vi "XY Graph Set Style of Selected Plots.vi"(8 "Error In":errorcluster, 9 "Plot Style":T2={"Plot Style"=enum."unchanged", "Histogram Type"=enum."Left Bound", "Line Tickness"=enum."unchanged", "Line Style"=enum."unchanged", "Point Style"=enum."Small Filled Square", "Line Color"=0, "Point Color"=0, "Anti-aliased"=FALSE, "Line Color Chooser"=enum."unchanged", "Point Color Chooser"=enum."unchanged", "Line Color List"="", "Point Color List"=""}, 11 "XYGraph Ref":T1) -> (0 "Error Out":errorcluster, 1 "Message":string, 3 "XYGraph Ref":T1, 5 "Graph Caption or Label":string)   [LabVIEW 2021, in "XY Graph Add-Ons.lvlib"]
uses:
  XY Graph Add-Ons.lvlib
  XY Graph Refnum.ctl
  Plot Style 3.ctl
  Graphs.lvlib
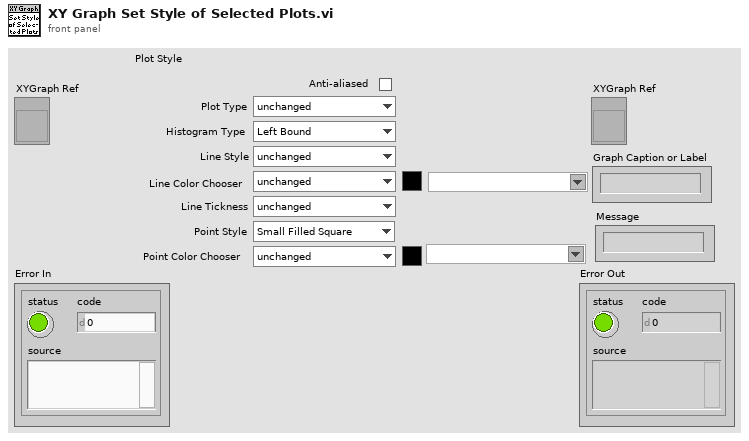
[diagram p1: front panel]
types:
  T1 = typedef "XY Graph Add-Ons.lvlib/XY Graph Refnum.ctl" = refnum<vi>
  T2 = typedef "Graphs.lvlib/Plot Style 3.ctl" = cluster{"Plot Style":enum16{"unchanged", "Line", "Symbol", "Line + Symbol", "Histogram", "Histogram + Symbol"}, "Histogram Type":enum16{"unchanged", "Left Bound", "Center", "Right Bound"}, "Line Tickness":enum16{"unchanged", "Thin", "1 pixel", "2 pixel", "3 pixel", "4 pixel", "5 pixel"}, "Line Style":enum16{"unchanged", "Plain", "Long Dash", "Short Dash", "Long-Short Dash", "Long-Short-Short Dash"}, "Point Style":enum16{"unchanged", "None", "Empty Circle", "Filled Circle", "Thick Circle", "Dotted Circle", "Empty Square", "Filled Square", "Thick Square", "Dotted Square", "Small Filled Square", "Dot", "Cross", "Tiny Cross", "Large X", "Small x", "Diamond", "Small Empty Square"}, "Line Color":u32, "Point Color":u32, "Anti-aliased":bool, "Line Color Chooser":enum16{"unchanged", "Color Box", "Color List"}, "Point Color Chooser":enum16{"unchanged", "Color Box", "Color List"}, "Line Color List":string, "Point Color List":string}
  T3 = typedef "Graphs.lvlib/Single Plot Style 2.ctl" = cluster{"Plot Style":enum16{"unchanged", "Line", "Symbol", "Line + Symbol", "Histogram", "Histogram + Symbol"}, "Histogram Type":enum16{"unchanged", "Left Bound", "Center", "Right Bound"}, "Line Tickness":enum16{"unchanged", "Thin", "1 pixel", "2 pixel", "3 pixel", "4 pixel", "5 pixel"}, "Line Style":enum16{"unchanged", "Plain", "Long Dash", "Short Dash", "Long-Short Dash", "Long-Short-Short Dash"}, "Point Style":enum16{"unchanged", "None", "Empty Circle", "Filled Circle", "Thick Circle", "Dotted Circle", "Empty Square", "Filled Square", "Thick Square", "Dotted Square", "Small Filled Square", "Dot", "Cross", "Tiny Cross", "Large X", "Small x", "Diamond", "Small Empty Square"}, "Line Color":u32, "Line Color defined?":bool, "Point Color":u32, "Point Color defined?":bool, "Anti-aliased":bool}
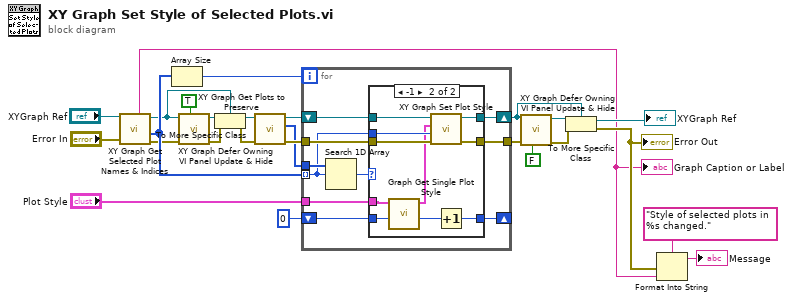
[diagram p0: block diagram]
diagram:
  n1 = call "XY Graph Get Selected Plot Names & Indices.vi"("error in (no error)"="Error In", "XYGraph in"="XYGraph Ref") -> ("error out"=w21:errorcluster, "Selected Plots"=w25:i32[], "XYGraph out"=w12:T1, "Graph Name"=w1:string)  [unwired: 5 in, 1 out]
  "Graph Caption or Label" <- w1
  n2 = Array Size(array=w25) -> (size(s)=w24:i32)
  n3 = call "XY Graph Defer Owning VI Panel Update & Hide.vi"("Defer Owning Panel Update"=TRUE, "error in (no error)"=w21, "XY Graph Refnum in"=w12) -> ("error out"=w11:errorcluster)  [unwired: 7 in, 1 out]
  n4 = To More Specific Class(target class=w12, reference=w12, error in=w11) -> (specific class reference=w7:T1, error out=w6:errorcluster)
  n5 = call "XY Graph Get Plots to Preserve.vi"("Error In"=w6, "XYGraph in"=w7) -> ("Error Out"=w5:errorcluster, "Preserved Plots"=w3:i32[], "XYGraph dup"=w4:T1)  [unwired: 6 in, 1 out]
  n6 = for {
    N: w24 -> [_]
    tunnel: w3 -> [w31]
    tunnel: w25 -> [w30] mode=indexing
    tunnel: "Plot Style" -> [w34]
    tunnel: w5 -> [w33]
    tunnel: [w32] -> w19
    shift-right: [w28] -> w9
    shift-left: w4 -> [w29]
    shift-right: [w26] -> _
    shift-left: 0 -> [w27]
    n7 = Search 1D Array(1D array=w31, element=w30) -> (index of element=w35:i32)  [unwired: 1 in]
    n8 = case shown="-1" w35 {
      tunnel: w30 -> [_ w43]
      tunnel: w29 -> [w37 w47]
      tunnel: w34 -> [_ w46]
      tunnel: w33 -> [w38 w45]
      tunnel: [w38 w44] -> w32
      tunnel: w27 -> [w36 w40]
      tunnel: [w37 w41] -> w28
      tunnel: [w36 w39] -> w26
      frame 0, Default {
      }
      frame -1 {
        n9 = call "Graph Get Single Plot Style.vi"("index"=w40, "Plot Style in"=w46) -> ("Plot Style out"=w42:T3)  [unwired: 8 in, 1 out]
        n10 = call "XY Graph Set Plot Style.vi"("Error In"=w45, "Plot Index (0)"=w43, "Single Plot Style"=w42, "XY Graph Refnum in"=w47) -> ("Error Out"=w44:errorcluster, "XY Graph Refnum out"=w41:T1)  [unwired: 6 in]
        n11 = Increment(x=w40) -> (x+1=w39:i32)
      }
    }
  }
  n12 = call "XY Graph Defer Owning VI Panel Update & Hide.vi"("Defer Owning Panel Update"=FALSE, "error in (no error)"=w19, "XY Graph Refnum in"=w9) -> ("error out"=w8:errorcluster, "XY Graph Refnum out"=w10:refnum<vi>)  [unwired: 7 in]
  n13 = To More Specific Class(target class=w9, reference=w10, error in=w8) -> (specific class reference=→"XYGraph Ref":T1, error out=w17:errorcluster)
  "Error Out" <- w17
  n14 = Format Into String(format string="Style of selected plots in %s changed.", error in=w17, w1) -> (resulting string=→"Message":string)  [unwired: 1 in, 1 out]
